vi "Control.AnalysisStart.vi"(11 "Parameters":T1={"Results Path"=path "C:/testdata/Logs", "Temp Path"=path "C:/testdata/Temp", "Remote Path"=path "d:/testdata/Logs", "Analysis VIs"=[], "Report Passed?"=FALSE, "Group Channels?"=FALSE}) -> (0 "error out":errorcluster, 3 "AnalysisRef":refnum<vi>)   [LabVIEW 2015, in "NIAnalysis.lvlib"]
uses:
  NIAnalysis.lvlib
  Types/AnalysisGUI.Parameters.ctl
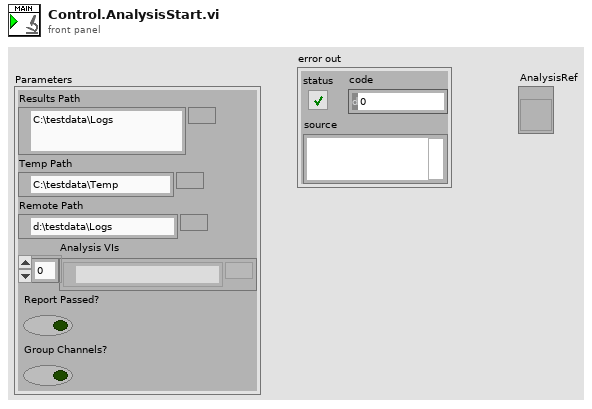
[diagram p1: front panel]
types:
  T1 = typedef "NIAnalysis.lvlib/AnalysisGUI.Parameters.ctl" = cluster{"Results Path":path, "Temp Path":path, "Remote Path":path, "Analysis VIs":path[], "Report Passed?":bool, "Group Channels?":bool}
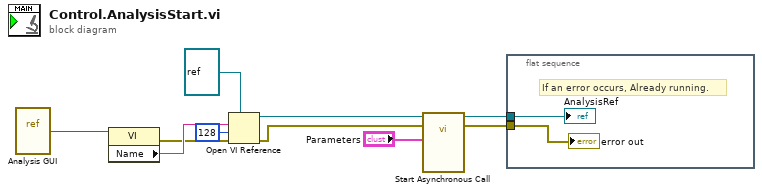
[diagram p0: block diagram]
diagram:
  n1 = vi-ref "Analysis GUI.vi"() -> (w10:refnum<vi>)
  n2 = property class="VI"(reference=w10) -> (error out=w4:errorcluster, "Name"=w9:string)  [unwired: 1 in, 1 out]
  n3 = Open VI Reference(type specifier VI Refnum (for type only)=refnum<vi> refnum, vi path=w9, options=128, error in (no error)=w4) -> (vi reference=w8:refnum<vi>, error out=w6:errorcluster)  [unwired: 2 in]
  n4 = call-by-ref "Start Asynchronous Call"(reference=w8, error in=w6, "Parameters"="Parameters") -> (reference out=w3:refnum<vi>, error out=w2:errorcluster)  [unwired: 11 in]
  n5 = flat-sequence {
    tunnel: w3 -> [w12]
    tunnel: w2 -> [w11]
    frame #0 {
      # "If an error occurs, Already running."
      "AnalysisRef" <- w12
      "error out" <- w11
    }
  }
